vi "Wait on Notifier.vi"(8 "Error In":errorcluster, 9 "timeout in ms (-1)":i32, 11 "notifier in":refnum<notifier>) -> (0 "Error Out":errorcluster, 1 "Data":variant, 3 "notifier out":refnum<notifier>)   [LabVIEW 2019, in "Data and Error Notifier.lvlib"]
uses:
  Data and Error Notifier.lvlib
  Data Error cluster.ctl
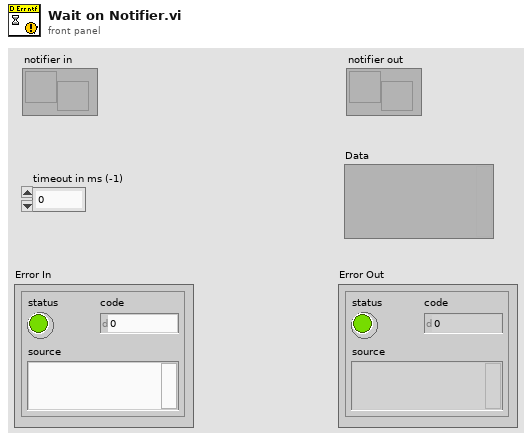
[diagram p1: front panel]
types:
  T1 = typedef "Data and Error Notifier.lvlib/Data Error cluster.ctl" = cluster{"Data":variant, "Error":errorcluster}
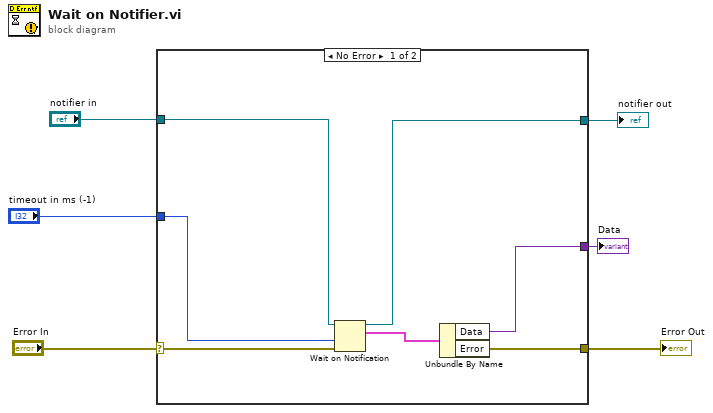
[diagram p0: block diagram]
diagram:
  n1 = case shown="No Error" "Error In" {
    selector: "Error In" -> [w13 w14]
    tunnel: [w8 w14] -> w5
    tunnel: [w12 _] -> w2
    tunnel: "timeout in ms (-1)" -> [w11 _]
    tunnel: "notifier in" -> [w10 _]
    tunnel: [w7 _] -> w1
    frame No Error {
      n2 = Wait on Notification(notifier=w10, timeout in ms (-1)=w11, error in (no error)=w13) -> (notifier out=w12:refnum<notifier>, notification=w9:T1)  [unwired: 1 in, 2 out]
      n3 = Unbundle By Name(w9) -> ("Data"=w7:variant, "Error"=w8:errorcluster)
    }
    frame Error {
    }
  }
  "Error Out" <- w5
  "notifier out" <- w2
  "Data" <- w1
